vi "Test - Relink Packages E2E.vi"() -> ()   [LabVIEW 2026]
doc: "Test harness: runs Relink Packages.vi over the disposable copies in C:\\Temp\\lvpm-test and exposes its results."
panel:
  out "Completed OK":bool
  out "error out":errorcluster
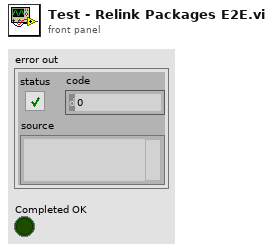
[diagram p1: front panel]
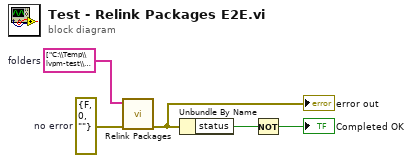
[diagram p0: block diagram]
diagram:
  w4 = errorcluster {"status"=FALSE, "code"=0, "source"=""}  # no error
  w5 = string[] ["C:\\Temp\\lvpm-test\\lunit", "C:\\Temp\\lvpm-test\\HSE Layout Manager"]  # folders
  n1 = call "Relink Packages.vi"("error in (no error)"=w4, "Folders to relink"=w5) -> ("error out"=w3:errorcluster)  [unwired: 9 in]
  "error out" <- w3
  n2 = Unbundle By Name(w3) -> ("status"=w2:bool)
  n3 = Not(x=w2) -> (.not. x?=→"Completed OK":bool)
